vi "Start Z stack.vi"(8 "error in (no error)":errorcluster, 10 "Camera Settings":T1={"Exposure Time (ms)"=100.0, "Binning"=enum."2x2", "Scan Mode"=0, "Frames to Acquire"=1000.0, "Pixel Correction"=TRUE, "Frames to Skip"=0, "File Path"=path "", "Duty cycle"=0.2, "ALEX"=FALSE, "Shutter Enable"=[], "fluidics trigger frame"=0, "Bit Depth"=0, "Image Width (px)"=0, "Image Height (px)"=0, "Horizontal Offset (px)"=0, "Vertical Offset (px)"=0} {"fluidics trigger frame" max=60000 step=1; "Exposure Time (ms)" min=1.0 max=10000.0 step=1.0}, 11 "Application in":refnum<class "Application.lvclass">) -> (0 "error out":errorcluster, 3 "Application out":refnum<class "Application.lvclass">)   [LabVIEW 2023, in "Application.lvlib" / "Application.lvclass"]
uses:
  Application.lvclass
  C:/Program Files/National Instruments/LabVIEW 2023/vi.lib/ActorFramework/Actor/Actor.lvclass
  Resources/Type Defs/Camera Settings.ctl
  Application.lvclass/Application.ctl
  Mode.ctl
  <vilib>/ActorFramework/Message Enqueuer/Message Enqueuer.lvclass/Message Enqueuer.ctl
  <vilib>/ActorFramework/Actor/Actor.lvclass/Actor.ctl
  Application Messages/Stop Live Mode Msg/Stop Live Mode Msg.lvclass/Stop Live Mode Msg.ctl
  Application Messages/Start Z stack Msg/Start Z stack Msg.lvclass/Start Z stack Msg.ctl
  <vilib>/ActorFramework/Message Enqueuer/Enqueue.vi
  <vilib>/ActorFramework/Message Enqueuer/Init from Existing Queue.vi
  Hardware/Stage Controller Messages/Start Autofocus Msg/Start Autofocus Msg.lvclass
  C:/Program Files/National Instruments/LabVIEW 2023/vi.lib/ActorFramework/Message/Message.lvclass
  Application Messages/Stop Live Mode Msg/Stop Live Mode Msg.lvclass
  Application Messages/Start Z stack Msg/Start Z stack Msg.lvclass
  <vilib>/ActorFramework/Message Priority Queue/Priority Enqueue.vi
  <vilib>/ActorFramework/Message Enqueuer/Message Enqueuer.lvclass
  Application.lvlib
  <vilib>/ActorFramework/Actor/Actor.lvclass
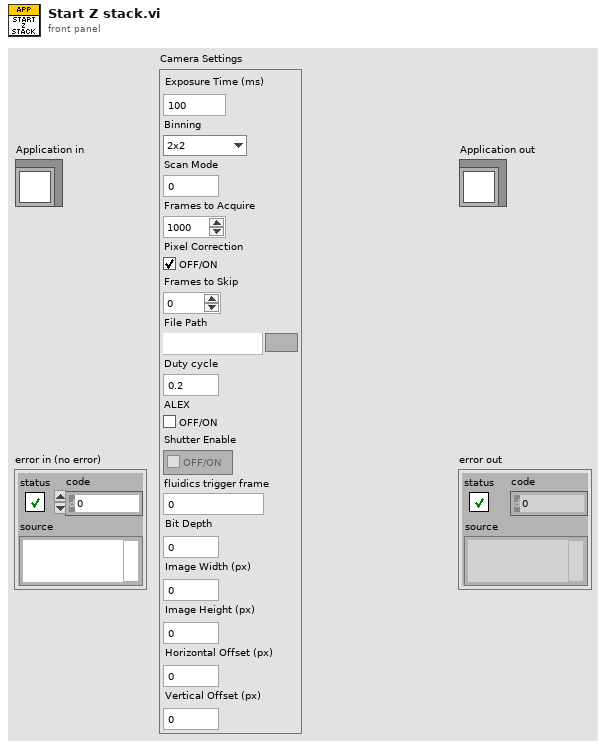
[diagram p1: front panel]
types:
  T1 = typedef "Camera Settings.ctl" = cluster{"Exposure Time (ms)":dbl, "Binning":enum16{"1x1", "2x2", "4x4"}, "Scan Mode":i32, "Frames to Acquire":dbl, "Pixel Correction":bool, "Frames to Skip":u32, "File Path":path, "Duty cycle":dbl, "ALEX":bool, "Shutter Enable":bool[], "fluidics trigger frame":u16, "Bit Depth":u16, "Image Width (px)":u16, "Image Height (px)":u16, "Horizontal Offset (px)":u16, "Vertical Offset (px)":u16}
  T2 = typedef "Application.lvlib/Mode.ctl" = enum16{"Idle", "Cancel", "Live", "Stream", "Autofocus", "Z-Stack", "Montage"}
  T3 = enum16{"Disabled", "ESP301", "Ti2", "Ludl", "ASI"}
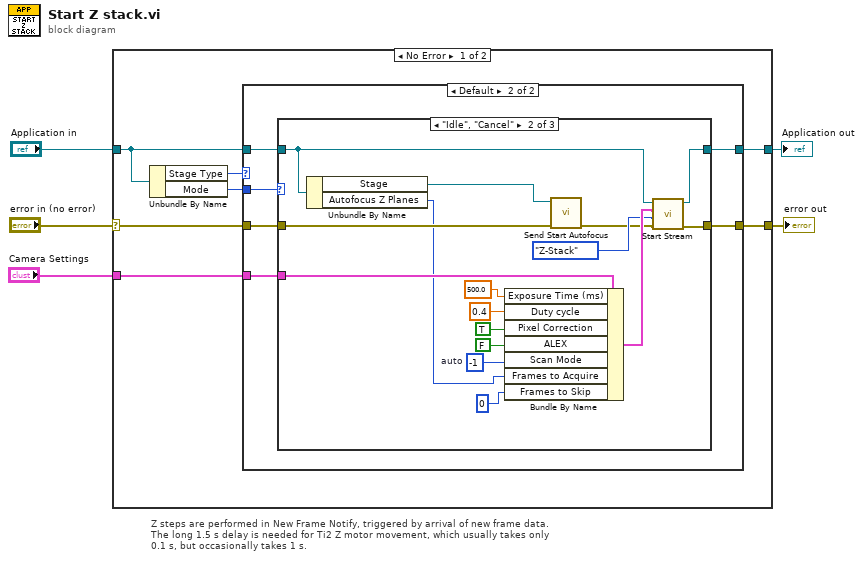
[diagram p0: block diagram]
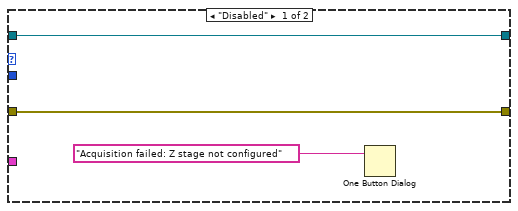
[diagram p2: hidden frame]
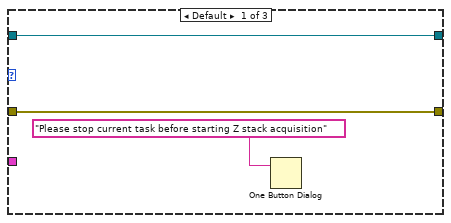
[diagram p3: hidden frame]
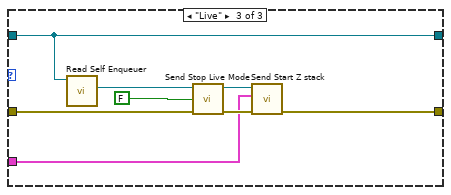
[diagram p4: hidden frame]
diagram:
  # "Z steps are performed in New Frame Notify, triggered by arrival of new frame data.\nThe long 1.5 s delay is needed for Ti2 Z motor movement, which usually takes only\n0.1 s, but occasionally takes 1 s."
  n1 = case shown="No Error" "error in (no error)" {
    selector: "error in (no error)" -> [w9 w50]
    tunnel: [w12 w50] -> w4
    tunnel: "Application in" -> [w7 w49]
    tunnel: "Camera Settings" -> [w10 _]
    tunnel: [w11 w49] -> w1
    frame No Error {
      n2 = Unbundle By Name(w7) -> ("Stage Type"=w8:T3, "Mode"=w6:T2)
      n3 = case shown="Default" w8 {
        tunnel: [w14 w21] -> w12
        tunnel: [w15 w20] -> w11
        tunnel: w10 -> [_ w19]
        tunnel: w9 -> [w14 w18]
        tunnel: w7 -> [w15 w17]
        tunnel: w6 -> [_ w16]
        frame "Disabled" {
          n4 = One Button Dialog(message="Acquisition failed: Z stage not configured") -> ()  [unwired: 1 in, 1 out]
        }
        frame Default {
          n5 = case shown="\"Idle\", \"Cancel\"" w16 {
            tunnel: [w23 w32 w43] -> w21
            tunnel: [w24 w31 w46] -> w20
            tunnel: w19 -> [_ w37 w41]
            tunnel: w18 -> [w23 w38 w45]
            tunnel: w17 -> [w24 w30 w46]
            frame Default {
              n6 = One Button Dialog(message="Please stop current task before starting Z stack acquisition") -> ()  [unwired: 1 in, 1 out]
            }
            frame "Idle", "Cancel" {
              w33 = -1  # auto
              n7 = Unbundle By Name(w30) -> ("Stage"=w35:refnum<class "Message Enqueuer.lvclass">, "Autofocus Z Planes"=w25:i32)
              n8 = Bundle By Name(cluster=w37, "Exposure Time (ms)"=500.0 ("frame interval (ms)"), "Duty cycle"=0.4, "Pixel Correction"=TRUE, "ALEX"=FALSE, "Scan Mode"=w33, "Frames to Acquire"=w25, "Frames to Skip"=u32 0) -> (w29:T1)
              n9 = call "Send Start Autofocus.vi"("error in (no error)"=w38, "Message Enqueuer"=w35) -> ("error out"=w27:errorcluster)  [unwired: 8 in, 1 out]
              n10 = call-dynamic "Start Stream.vi"("error in (no error)"=w27, "Mode"=Mode."Z-Stack", "Camera Settings"=w29, "Application in"=w30) -> ("error out"=w32:errorcluster, "Application out"=w31:refnum<class "Application.lvclass">)  [unwired: 6 in]
            }
            frame "Live" {
              n11 = call <vilib>:"Read Self Enqueuer.vi"("Actor"=w46) -> ("Self Enqueuer"=w47:refnum<class "Message Enqueuer.lvclass">)  [unwired: 10 in]
              n12 = call "Send Stop Live Mode.vi"("error in (no error)"=w45, "Close Viewer"=FALSE, "Message Enqueuer"=w47) -> ("error out"=w44:errorcluster, "Message Enqueuer out"=w42:refnum<class "Message Enqueuer.lvclass">)  [unwired: 7 in]
              n13 = call "Send Start Z stack.vi"("error in (no error)"=w44, "Camera Settings"=w41, "Message Enqueuer"=w42) -> ("error out"=w43:errorcluster)  [unwired: 7 in, 1 out]
            }
          }
        }
      }
    }
    frame Error {
    }
  }
  "error out" <- w4
  "Application out" <- w1
